vi "Actor Core.vi"(8 "error in":errorcluster, 11 "PLCHandler in":refnum<class "PLCHandler.lvclass">) -> (0 "error out":errorcluster, 3 "Actor out":refnum<class "Actor.lvclass">)   [LabVIEW 2022 SP3, in "PLCHandler.lvlib" / "PLCHandler.lvclass"]
doc: "(<B>Filename</B>: Actor Framework.lvlib:Actor.lvclass:Actor Core.vi)\n\nReceives messages to the actor, reacts to them, and initiates any error handling that may shut the actor down.\n\nDescendant classes may override this VI to append parallel tasks for the actor to complete while it handles messages. Overrides use the Call Parent Class Method node."
uses:
  PLCHandler.lvclass
  C:/Program Files/National Instruments/LabVIEW 2022/vi.lib/ActorFramework/Actor/Actor.lvclass
  <vilib>/ActorFramework/Actor/Actor.lvclass
  PLCHandler.lvclass/PLCHandler.ctl
  <vilib>/ActorFramework/Actor/Actor.lvclass/Actor.ctl
  <vilib>/ActorFramework/Message Enqueuer/Message Enqueuer.lvclass/Message Enqueuer.ctl
  <vilib>/ActorFramework/Message Enqueuer/Init from Existing Queue.vi
  <vilib>/ActorFramework/Message Enqueuer/Enqueue.vi
  PLCHandler - Controller -- Interface/PLCHandler - Controller -- Interface Messages/Image Request Msg/Image Request Msg.lvclass
  C:/Program Files/National Instruments/LabVIEW 2022/vi.lib/ActorFramework/Message/Message.lvclass
  <vilib>/ActorFramework/Message Priority Queue/Priority Enqueue.vi
  <vilib>/ActorFramework/Message Enqueuer/Message Enqueuer.lvclass
  <vilib>/NI/Modbus Library/API/Master/Modbus Master.lvclass
  E:/GitHub/image-harvest/PLCHandler/PLCHandler/PLCHandler.lvclass
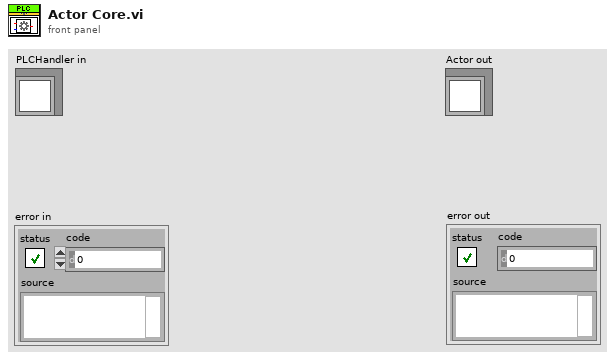
[diagram p1: front panel]
types:
  T1 = cluster{"Ack":refnum<user-event>, "Stop":refnum<user-event>, "Awake":refnum<user-event>}
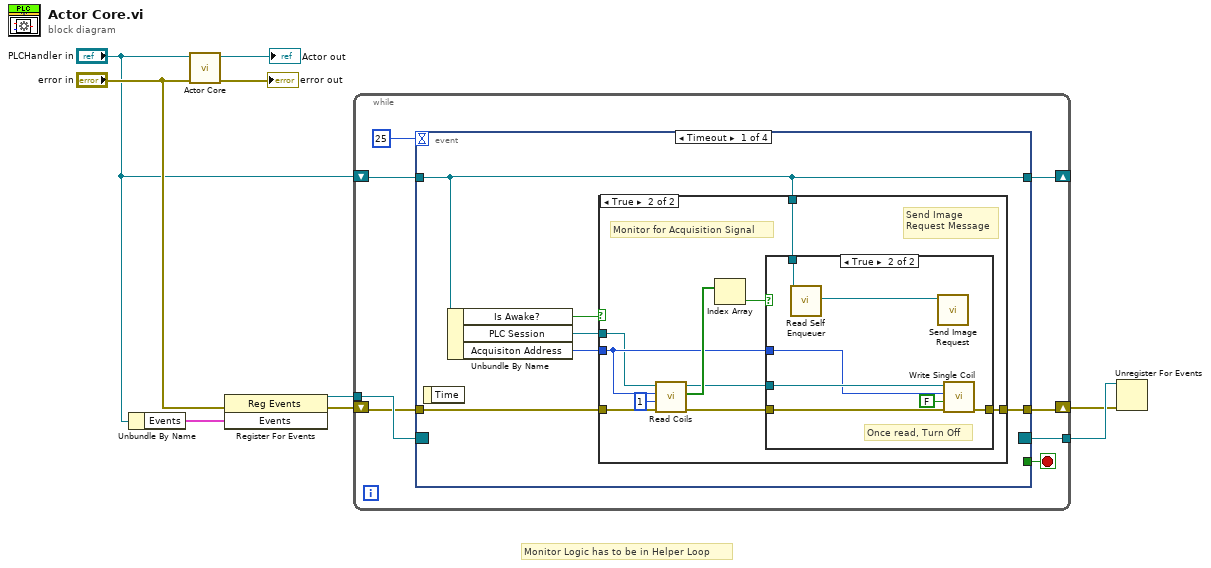
[diagram p0: block diagram]
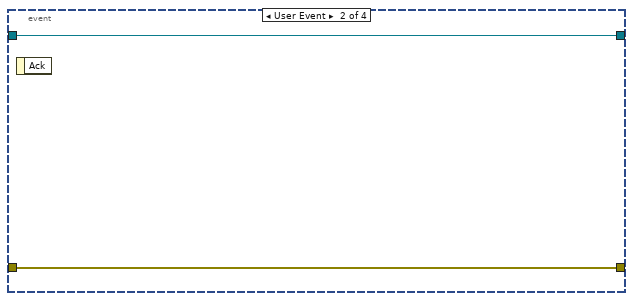
[diagram p4: hidden frame]
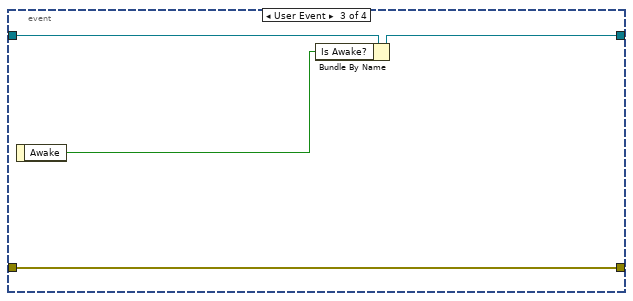
[diagram p5: hidden frame]
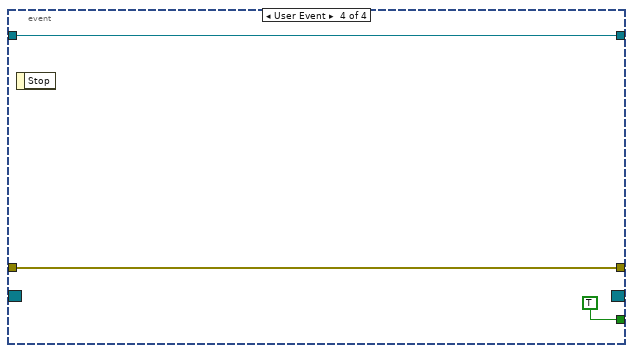
[diagram p6: hidden frame]
diagram:
  # "Monitor Logic has to be in Helper Loop"
  n1 = Unbundle By Name("PLCHandler in") -> ("Events"=w1:T1)
  n2 = call-parent "Actor Core.vi"("error in"="error in", "Actor in"="PLCHandler in") -> ("error out"=→"error out":errorcluster, "Actor out"=→"Actor out":refnum<class "Actor.lvclass">)  [unwired: 8 in]
  n3 = register-events(error in="error in", w1) -> (reference out=w4:refnum<event-registration>, error out=w7:errorcluster)  [unwired: 1 in]
  n4 = while {
    shift-right: [w16] -> _
    shift-left: "PLCHandler in" -> [w17]
    shift-right: [w11] -> w2
    shift-left: w7 -> [w12]
    tunnel: w4 -> [w15]
    tunnel: [w10] -> w3
    stop <- w13 stop-if-true
    n5 = event shown="[0] Timeout" {
      selector: w15 -> [_ _ _ _]
      dyn-events: [_ _ _ _] -> w10
      timeout: 25 -> [_ _ _ _]
      tunnel: w17 -> [w21 w44 w48 w50]
      tunnel: [w21 w44 w47 w50] -> w16
      tunnel: [_ _ _ TRUE] -> w13
      tunnel: w12 -> [w23 w43 w45 w49]
      tunnel: [w22 w43 w45 w49] -> w11
      event Timeout {
        n6 = event-data() -> ()  [unwired: 1 in, 1 out]
        n7 = Unbundle By Name(w21) -> ("Is Awake?"=w18:bool, "PLC Session"=w19:refnum<class "Modbus Master.lvclass">, "Acquisiton Address"=w20:u16)
        n8 = case shown="True" w18 {
          tunnel: w23 -> [w24 w34]
          tunnel: [w24 w29] -> w22
          tunnel: w21 -> [_ w27]
          tunnel: w20 -> [_ w26]
          tunnel: w19 -> [_ w25]
          frame False {
            # "Waiting for Wakeup Signal"
          }
          frame True {
            # "Monitor for Acquisition Signal"
            # "Send Image\nRequest Message"
            n9 = call-dynamic "Read Coils.vi"("error in"=w34, "number of inputs"=u16 1, "starting address"=w26, "Modbus master in"=w25) -> ("error out"=w30:errorcluster, "coils"=w32:bool[], "Modbus master out"=w28:refnum<class "Modbus Master.lvclass">)  [unwired: 5 in]
            n10 = Index Array(array=w32) -> (element=w31:bool)  [unwired: 1 in]
            n11 = case shown="True" w31 {
              tunnel: w27 -> [_ w42]
              tunnel: w30 -> [w35 w41]
              tunnel: [w35 w40] -> w29
              tunnel: w28 -> [_ w39]
              tunnel: w26 -> [_ w37]
              frame False {
              }
              frame True {
                # "Once read, Turn Off"
                n12 = call <vilib>:"Read Self Enqueuer.vi"("Actor"=w42) -> ("Self Enqueuer"=w36:refnum<class "Message Enqueuer.lvclass">)  [unwired: 10 in]
                n13 = call "Send Image Request.vi"("Message Enqueuer"=w36) -> ()  [unwired: 9 in, 2 out]
                n14 = call-dynamic "Write Single Coil.vi"("error in"=w41, "coil to write"=FALSE, "address"=w37, "Modbus master in"=w39) -> ("error out"=w40:errorcluster)  [unwired: 6 in, 1 out]
              }
            }
          }
        }
      }
      event User Event {
        n15 = event-data() -> ()  [unwired: 1 in, 1 out]
      }
      event User Event {
        n16 = event-data() -> ("Awake"=w46:bool)  [unwired: 1 in]
        n17 = Bundle By Name(cluster=w48, "Is Awake?"=w46) -> (w47:refnum<class "PLCHandler.lvclass">)
      }
      event User Event {
        n18 = event-data() -> ()  [unwired: 1 in, 1 out]
      }
    }
  }
  n19 = Unregister For Events(event registration refnum=w3, error in=w2) -> ()  [unwired: 1 out]
